vi "Calc_focus.vi"(0 "Pos X":dbl, 1 "a0":dbl, 5 "Pos Y":dbl, 9 "Cen X":dbl, 11 "Cen Y":dbl, 12 "a1":dbl, 13 "a2":dbl, 14 "a3":dbl) -> (6 "Foyer":dbl, 10 "Residu":dbl)   [LabVIEW 2011]
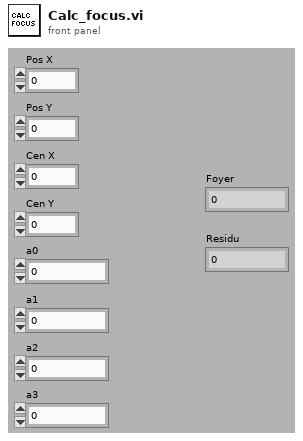
[diagram p1: front panel]
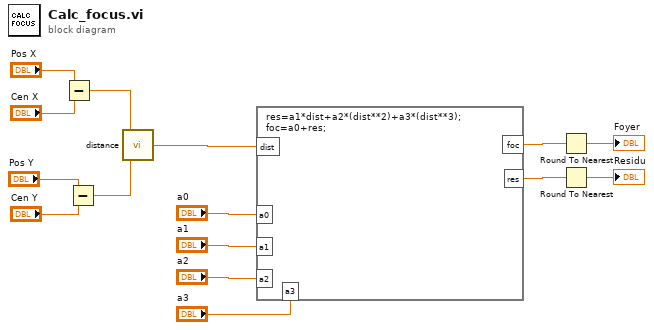
[diagram p0: block diagram]
diagram:
  n1 = Subtract(x="Pos X", y="Cen X") -> (x-y=w2:dbl)
  n2 = Subtract(x="Pos Y", y="Cen Y") -> (x-y=w3:dbl)
  n3 = call "distance.vi"("D2"=w3, "D1"=w2) -> ("DT"=w1:dbl)
  n4 = formula code="res=a1*dist+a2*(dist**2)+a3*(dist**3);\nfoc=a0+res;"("dist"=w1, "a0"="a0", "a1"="a1", "a2"="a2", "a3"="a3") -> ("foc"=w8:dbl, "res"=w6:dbl)
  n5 = Round To Nearest(number=w8) -> (nearest integer value=→"Foyer":dbl)
  n6 = Round To Nearest(number=w6) -> (nearest integer value=→"Residu":dbl)
